vi "Phasor Convert (m, phi) to (g,s).vi"(2 "Phasor (m, phi)":T1) -> (7 "Phasor (g, s)":T2)   [LabVIEW 2021, in "Phasor.lvlib"]
uses:
  Phasor.lvlib
  Phasor (g, s).ctl
  Phasor (m, phi).ctl
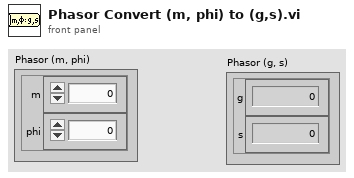
[diagram p1: front panel]
types:
  T1 = typedef "Phasor.lvlib/Phasor (m, phi).ctl" = cluster{"m":dbl, "phi":dbl}
  T2 = typedef "Phasor.lvlib/Phasor (g, s).ctl" = cluster{"g":dbl, "s":dbl}
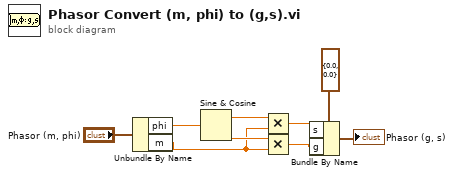
[diagram p0: block diagram]
diagram:
  n1 = Unbundle By Name("Phasor (m, phi)") -> ("phi"=w8:dbl, "m"=w3:dbl)
  n2 = Sine & Cosine(0:w8) -> (1:w7:dbl, 2:w4:dbl)
  n3 = Multiply(x=w7, y=w3) -> (x*y=w5:dbl)
  n4 = Multiply(x=w4, y=w3) -> (x*y=w2:dbl)
  n5 = Bundle By Name(cluster=T2 {"g"=0.0, "s"=0.0} ("Phasor (g, s)"), "s"=w5, "g"=w2) -> (→"Phasor (g, s)":T2)
